vi "Graph to Imaq Image 2010.vi"() -> ()   [LabVIEW 2010]
uses:
  <vilib>/vision/NI_Vision_Development_Module.lvlib
panel:
  out "Image":T1(plugin-control)
  in  "stop":bool
  out "Waveform Chart":i32(graph)
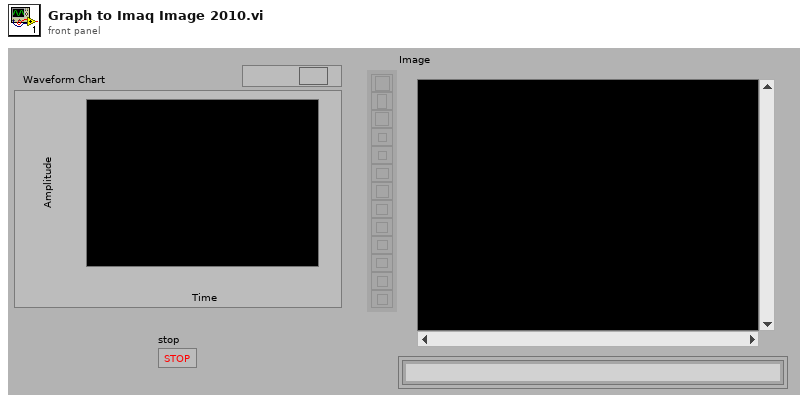
[diagram p1: front panel]
types:
  T1 = typedef "IMAQ Image.ctl" = refnum<image>
  T2 = typedef "Image Type" = u32
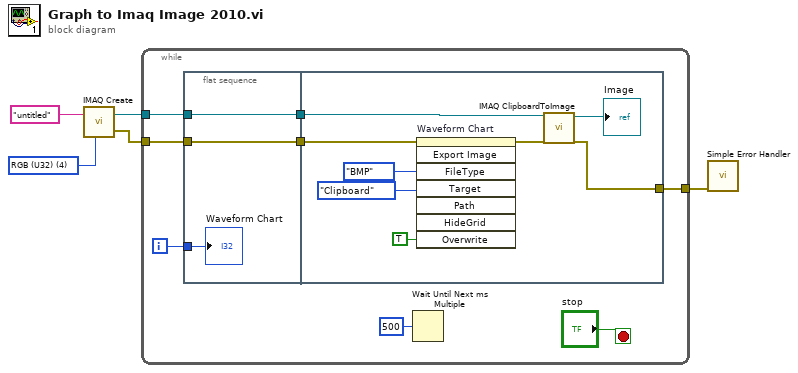
[diagram p0: block diagram]
diagram:
  w2 = T2 4 items=["Grayscale (U8)", "Grayscale (I16)", "Grayscale (SGL)", "Complex (CSG)", "RGB (U32)", "HSL (U32)", "RGB (U64)", "Grayscale (U16)"] ("Image Type")
  n1 = call "IMAQ Create"("Image Name"="untitled", "Image Type"=w2) -> ("New Image"=w4:T1, "error out"=w5:errorcluster)  [unwired: 3 in]
  n2 = while {
    tunnel: w5 -> [w10]
    tunnel: w4 -> [w12]
    tunnel: [w7] -> w1
    i -> [w8]
    stop <- "stop" stop-if-true
    n3 = flat-sequence {
      tunnel: w12 -> [w16]
      tunnel: [w16] -> w11
      tunnel: w10 -> [w15]
      tunnel: [w15] -> w9
      tunnel: w8 -> [w14]
      tunnel: w11 -> [w19]
      tunnel: w9 -> [w18]
      tunnel: [w17] -> w7
      frame #0 {
        "Waveform Chart" <- w14
      }
      frame #1 {
        n4 = invoke on="Waveform Chart" class="WFChart (strict)" method="Export Image"(error in=w18, "FileType"=enum32{"BMP", "EPS", "EMF", "PICT"}."BMP" ("File Type"), "Target"=enum32{"File", "Clipboard"}."Clipboard", "Overwrite"=TRUE ("Always Overwrite")) -> (error out=w20:errorcluster)  [unwired: 4 in, 7 out]
        n5 = call "IMAQ ClipboardToImage"("error in (no error)"=w20, "Image"=w19) -> ("error out"=w17:errorcluster, "Image Out"=→"Image":T1)  [unwired: 3 in, 2 out]
      }
    }
    n6 = Wait Until Next ms Multiple(millisecond multiple=u32 500) -> ()  [unwired: 1 out]
  }
  n7 = call <vilib>:"Simple Error Handler.vi"("error in (no error)"=w1) -> ()  [unwired: 4 in, 5 out]
